vi "niScope Reset with Defaults.vi"(0 "instrument handle":refnum<k15>, 11 "error in":errorcluster) -> (4 "instrument handle out":refnum<k15>, 15 "error out":errorcluster)   [LabVIEW 2011]
doc: "Resets the device to the default state and applies any initial default settings from the IVI Configuration Store. This VI uses default parameters to do a software reset on the device The changes are not immediately committed to hardware."
uses:
  niScope_32.dll
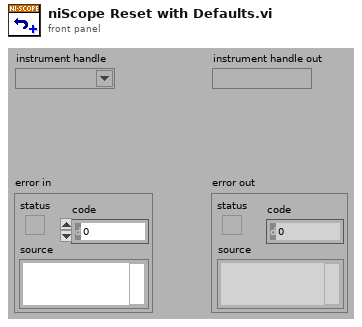
[diagram p1: front panel]
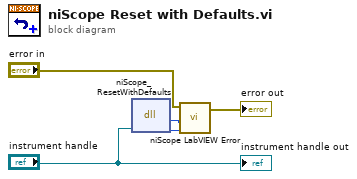
[diagram p0: block diagram]
diagram:
  n1 = dll-call lib="niScope_*.*" fn="niScope_ResetWithDefaults" ("niScope_reset")("instrumentHandle"="instrument handle") -> (w5:i32, "instrumentHandle"=w4:i32)  [unwired: 3 in, 2 out]
  n2 = call <instrlib>:"niScope LabVIEW Error.vi"("instrument handle"=w4, "niScope error code (0)"=w5, "error in (no error)"="error in") -> ("error out"=→"error out":errorcluster)  [unwired: 2 in]
  "instrument handle out" <- "instrument handle"
